vi "Modbus-Conversion.vi"(6 "Reg":dbl, 8 "error in (no error)":errorcluster, 9 "Scale Min range":dbl, 10 "Scale Max Range":dbl) -> (0 "error out":errorcluster, 2 "output":dbl)   [LabVIEW 2016]
panel:
  # "Formula node to calc the modbus Reg \nto real numbers.\nin the Adam 4000/5000 range modules."
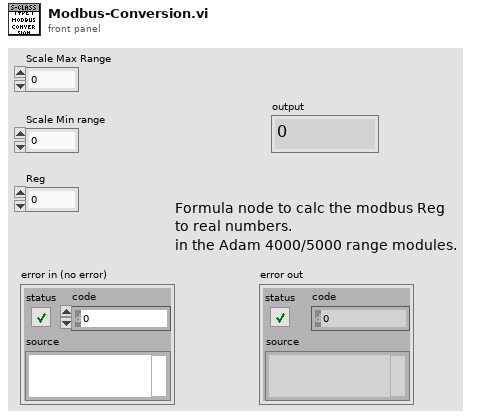
[diagram p1: front panel]
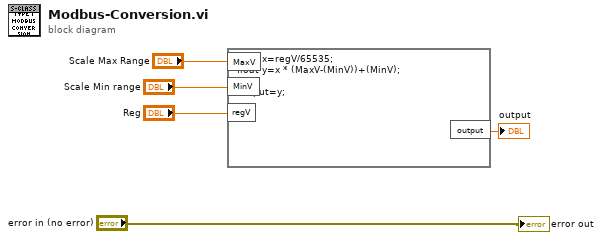
[diagram p0: block diagram]
diagram:
  n1 = formula code="float x=regV/65535;\nfloat y=x * (MaxV-(MinV))+(MinV);\n\noutput=y;"("MaxV"="Scale Max Range", "MinV"="Scale Min range", "regV"="Reg") -> ("output"=→"output":dbl)
  "error out" <- "error in (no error)"
